vi "ICM Create Scaling Table.vi"(8 "Instances":cluster{"Instances":string[]}[](array[cluster]), 9 "Scalings":string[](array[string]), 10 "Channels":string[](array[string]), 11 "Scalings In":T1[](array[typedef])) -> (3 "Table":string[][](array[string]))   [LabVIEW 2024]
doc: "*.vi\n\nInstrument Communication Module Version 1.0\nJuly, 2017 Original Code Consulting David Thomson\n www.originalcode.com"
uses:
  Scaling/Scaling Def.ctl
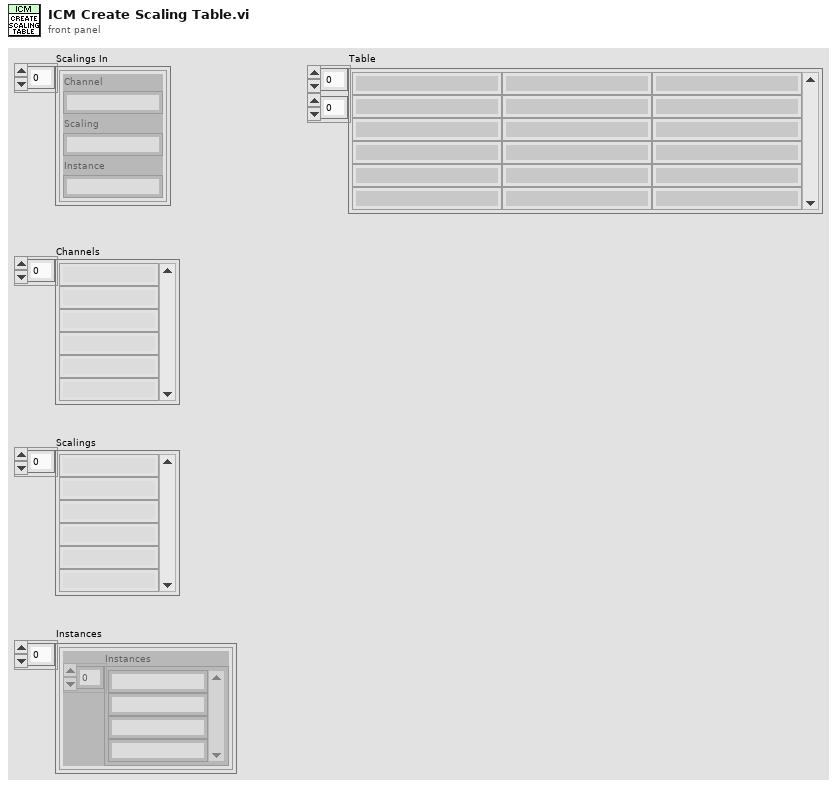
[diagram p1: front panel]
types:
  T1 = typedef "Scaling Def.ctl" = cluster{"Channel":string, "Scaling":string, "Instance":string}
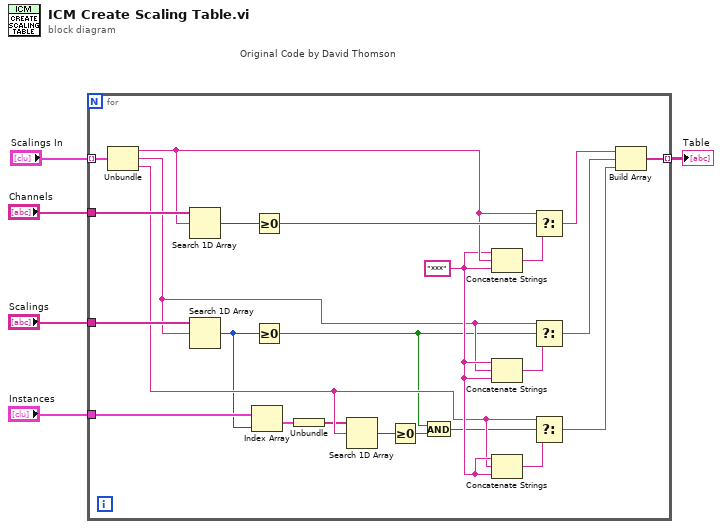
[diagram p0: block diagram]
diagram:
  n1 = for "Original Code by David Thomson" {
    tunnel: "Scalings In" -> [w29] mode=indexing
    tunnel: [w28] -> w4 mode=indexing
    tunnel: "Channels" -> [w27]
    tunnel: "Scalings" -> [w18]
    tunnel: "Instances" -> [w13]
    w17 = "***" ("string")
    n2 = Unbundle(w29) -> ("Channel"=w23:string, "Scaling"=w16:string, "Instance"=w14:string)
    n3 = Search 1D Array(1D array=w27, element=w23) -> (index of element=w26:i32)  [unwired: 1 in]
    n4 = Search 1D Array(1D array=w18, element=w16) -> (index of element=w11:i32)  [unwired: 1 in]
    n5 = Index Array(array=w13, index=w11) -> (element=w15:cluster{"Instances":string[]})
    n6 = Greater Or Equal To 0?(x=w26) -> (x >= 0?=w25:bool)
    n7 = Greater Or Equal To 0?(x=w11) -> (x >= 0?=w8:bool)
    n8 = Unbundle(w15) -> ("Instances"=w12:string[])
    n9 = Search 1D Array(1D array=w12, element=w14) -> (index of element=w20:i32)  [unwired: 1 in]
    n10 = Greater Or Equal To 0?(x=w20) -> (x >= 0?=w10:bool)
    n11 = And(x=w8, y=w10) -> (x .and. y?=w9:bool)
    n12 = Concatenate Strings(w17, w23, w17) -> (w22:string)
    n13 = Concatenate Strings(w17, w16, w17) -> (w21:string)
    n14 = Concatenate Strings(w17, w14, w17) -> (w19:string)
    n15 = Select(t=w23, s=w25, f=w22) -> (s? t:f=w24:string)
    n16 = Select(t=w16, s=w8, f=w21) -> (s? t:f=w7:string)
    n17 = Select(t=w14, s=w9, f=w19) -> (s? t:f=w6:string)
    n18 = Build Array(w24, w7, w6) -> (w28:string[])
  }
  "Table" <- w4
